vi "BuildPathToDynamic.vi"(10 "target VI relative path":path) -> (2 "target VI absolute path":path)   [LabVIEW 2013, in "LVTM.lvlib"]
doc: "Builds the correct path to the disk folder where the dynamic (ACBR) VIs reside, regardless of the location of this VI's calling VI. This is necessary because the path will be different when run from a deployed toolkit, even though both scenarios are in development mode."
uses:
  LVTM.lvlib
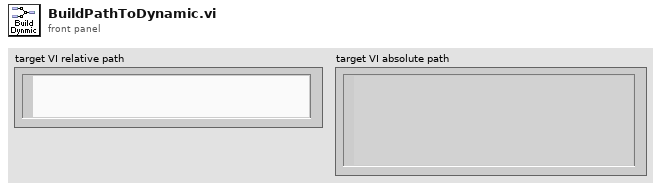
[diagram p1: front panel]
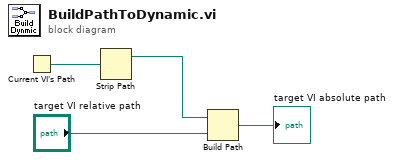
[diagram p0: block diagram]
diagram:
  n1 = Current VI's Path() -> (path=w4:path)
  n2 = Strip Path(path=w4) -> (stripped path=w1:path)  [unwired: 1 out]
  n3 = Build Path(base path=w1, name or relative path="target VI relative path") -> (appended path=→"target VI absolute path":path)
